vi "update Test.vi"(7 "Test.lvclass":refnum<class "Test.lvclass">, 8 "error in (no error)":errorcluster, 10 "index":i32 caption="Index", 11 "Report in":refnum<class "Report.lvclass">) -> (0 "error out":errorcluster, 3 "Report out":refnum<class "Report.lvclass">)   [LabVIEW 2013, in "DatenKlassen.lvlib" / "Report.lvclass"]
uses:
  Report.lvclass
  Test/Test.lvclass
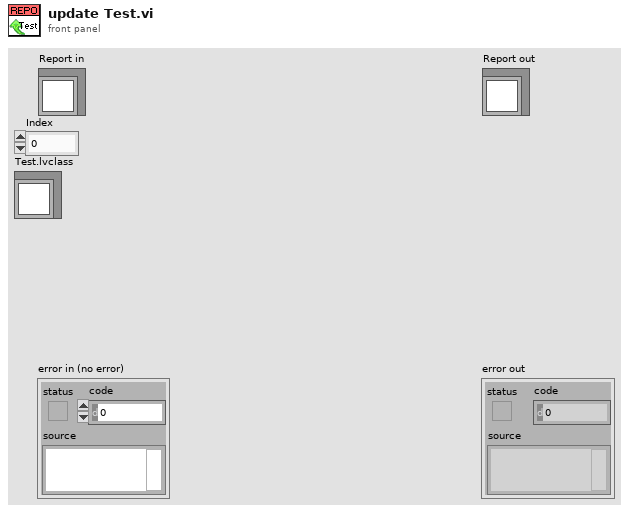
[diagram p1: front panel]
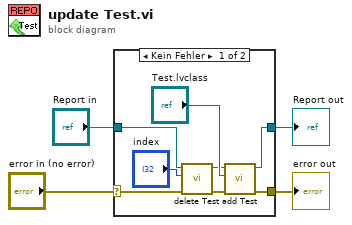
[diagram p0: block diagram]
diagram:
  n1 = case shown="Kein Fehler" "error in (no error)" {
    selector: "error in (no error)" -> [w10 w14]
    tunnel: [w5 w14] -> w3
    tunnel: [w6 w13] -> w1
    tunnel: "Report in" -> [w12 w13]
    frame No Error {
      n2 = call-dynamic "delete Test.vi"("error in (no error)"=w10, "index"="index", "Report (Eingang)"=w12) -> ("error out"=w7:errorcluster, "Report (Ausgang)"=w8:refnum<class "Report.lvclass">)  [unwired: 7 in]
      n3 = call-dynamic "add Test.vi"("error in (no error)"=w7, "Test.lvclass"="Test.lvclass", "Report (Eingang)"=w8) -> ("error out"=w5:errorcluster, "Report (Ausgang)"=w6:refnum<class "Report.lvclass">)  [unwired: 7 in]
    }
    frame Error {
    }
  }
  "error out" <- w3
  "Report out" <- w1
